vi "Tanget of Waypoint Segment.vi"(9 "point c":cluster{"x":dbl, "y":dbl}, 10 "point b":cluster{"x":dbl, "y":dbl}, 11 "point a":cluster{"x":dbl, "y":dbl}) -> (3 "T_i":cluster{dbl, dbl})   [LabVIEW 2019]
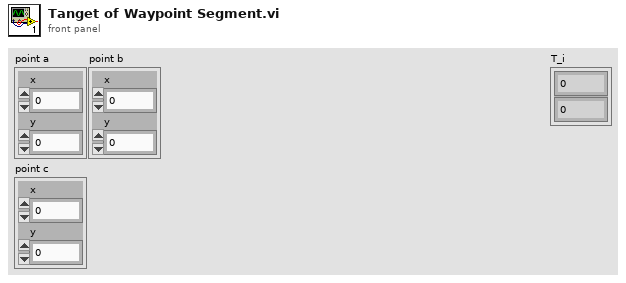
[diagram p1: front panel]
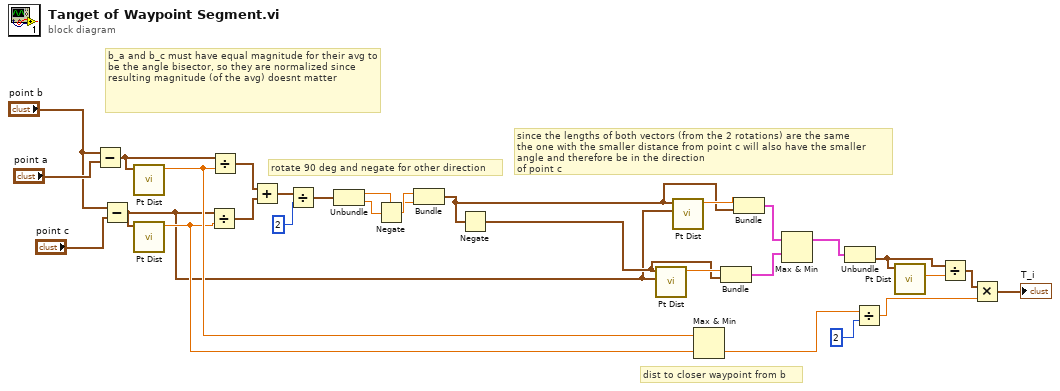
[diagram p0: block diagram]
diagram:
  # "b_a and b_c must have equal magnitude for their avg to be the angle bisector, so they are normalized since resulting magnitude (of the avg) doesnt matter"
  # "dist to closer waypoint from b"
  # "since the lengths of both vectors (from the 2 rotations) are the same\nthe one with the smaller distance from point c will also have the smaller angle and therefore be in the direction\nof point c"
  # "rotate 90 deg and negate for other direction"
  n1 = Subtract(x="point b", y="point a") -> (x-y=w28:cluster{"x":dbl, "y":dbl})
  n2 = Subtract(x="point b", y="point c") -> (x-y=w4:cluster{"x":dbl, "y":dbl})
  n3 = call "Pt Dist.vi"("point a"=w28) -> ("dist"=w12:dbl)  [unwired: 10 in]
  n4 = call "Pt Dist.vi"("point a"=w4) -> ("dist"=w11:dbl)  [unwired: 10 in]
  n5 = Divide(x=w4, y=w11) -> (x/y=w26:cluster{"x":dbl, "y":dbl})
  n6 = Divide(x=w28, y=w12) -> (x/y=w27:cluster{"x":dbl, "y":dbl})
  n7 = Add(x=w27, y=w26) -> (x+y=w25:cluster{"x":dbl, "y":dbl})
  n8 = Divide(x=w25, y=u16 2) -> (x/y=w23:cluster{"x":dbl, "y":dbl})
  n9 = Unbundle(w23) -> ("x"=w20:dbl, "y"=w22:dbl)
  n10 = Negate(x=w22) -> (-x=w21:dbl)
  n11 = Bundle(w21, "x"=w20) -> (w6:cluster{dbl, "x":dbl})  [unwired: 1 in]
  n12 = Negate(x=w6) -> (-x=w5:cluster{dbl, "x":dbl})
  n13 = call "Pt Dist.vi"("point b"=w4, "point a"=w5) -> ("dist"=w17:dbl)  [unwired: 9 in]
  n14 = call "Pt Dist.vi"("point b"=w4, "point a"=w6) -> ("dist"=w18:dbl)  [unwired: 9 in]
  n15 = Max & Min(x=w12, y=w11) -> (min(x,y)=w10:dbl)  [unwired: 1 out]
  n16 = Bundle("dist"=w17, w5) -> (w15:cluster{"dist":dbl, cluster{dbl, "x":dbl}})  [unwired: 1 in]
  n17 = Bundle("dist"=w18, w6) -> (w16:cluster{"dist":dbl, cluster{dbl, "x":dbl}})  [unwired: 1 in]
  n18 = Max & Min(x=w16, y=w15) -> (max(x,y)=w1:cluster{"dist":dbl, cluster{dbl, "x":dbl}})  [unwired: 1 out]
  n19 = Unbundle(w1) -> (w8:cluster{dbl, "x":dbl})  [unwired: 1 out]
  n20 = Divide(x=w10, y=u16 2) -> (x/y=w14:dbl)
  n21 = call "Pt Dist.vi"("point a"=w8) -> ("dist"=w9:dbl)  [unwired: 10 in]
  n22 = Divide(x=w8, y=w9) -> (x/y=w7:cluster{dbl, "x":dbl})
  n23 = Multiply(x=w7, y=w14) -> (x*y=→"T_i":cluster{dbl, "x":dbl})
